vi "TriangleContinuityTracepoint.vi"(7 "service name":string, 8 "error in (no error)":errorcluster, 9 "max difference":dbl, 10 "Acq Block Number":i32, 11 "Qbus in":refnum<class "Qbus.lvclass">) -> (0 "error out":errorcluster)   [LabVIEW 2015]
uses:
  <vilib>/addons/Qbus/Qbus.lvclass
  <vilib>/addons/TraceLogger/TraceLogger.lvlib
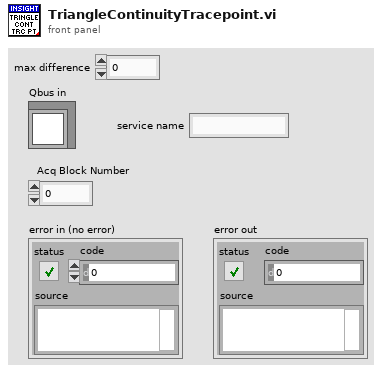
[diagram p1: front panel]
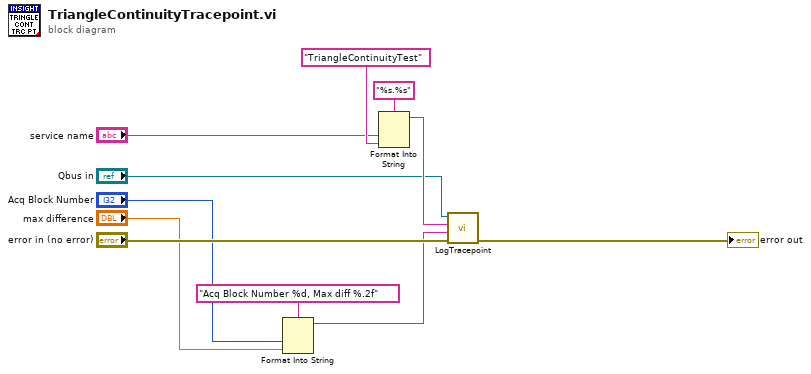
[diagram p0: block diagram]
diagram:
  n1 = Format Into String(format string="Acq Block Number %d, Max diff %.2f", "Acq Block Number", "max difference") -> (resulting string=w1:string)  [unwired: 2 in, 1 out]
  n2 = Format Into String(format string="%s.%s", "service name", "TriangleContinuityTest" ("tracepoint")) -> (resulting string=w8:string)  [unwired: 2 in, 1 out]
  n3 = call <vilib>:"LogTracepoint.vi"("error in (no error)"="error in (no error)", "log string"=w1, "tracepoint"=w8, "qbus in"="Qbus in") -> ("error out"=→"error out":errorcluster)  [unwired: 6 in, 1 out]
